vi "readFromXML.vi"(8 "error in (no error)":errorcluster, 10 "XML in":string, 11 "POrigin in":refnum<class "POrigin.lvclass">) -> (0 "error out":errorcluster, 3 "POrigin out":refnum<class "POrigin.lvclass">)   [LabVIEW 2022 SP3, in "TCSDataDefinitions.lvlib" / "TCSCommand.lvlib" / "POriginCommands.lvlib" / "POrigin.lvclass"]
uses:
  POrigin.lvclass
  <userlib>/Common/UnitsAndXML/FlattenItemWithUnitToXML/FlattenLengthToXML/LengthUnit.ctl
  POrigin.lvclass/POrigin.ctl
  POriginCommands/POriginCommands.lvclass
  <userlib>/Common/UnitsAndXML/UnitsAndXML.lvlib
  <userlib>/Common/XML/XMLParser/XMLParser.lvclass
panel:
  out "pOriginY":dbl[unit]
  out "pOriginX":dbl[unit]
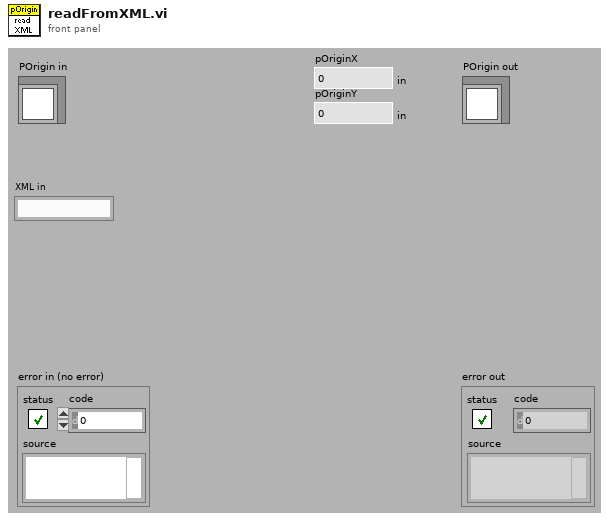
[diagram p1: front panel]
types:
  T1 = typedef "UnitsAndXML.lvlib/LengthUnit.ctl" = enum16{"m", "Angstrom", "AU", "chain", "cm", "cubit", "fathom", "fermi", "ft", "furlong", "hubble", "in", "ly", "mi", "mm", "rod", "um", "yd"}
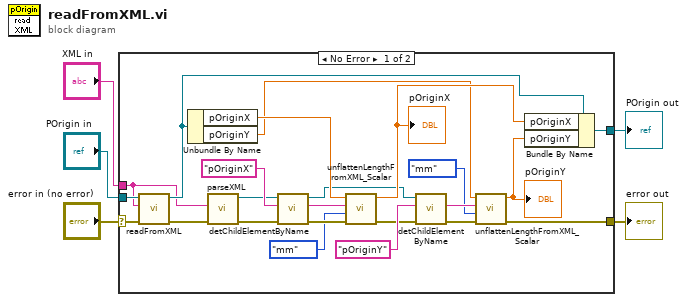
[diagram p0: block diagram]
diagram:
  n1 = case shown="No Error" "error in (no error)" {
    selector: "error in (no error)" -> [w22 w30]
    tunnel: [w8 w30] -> w4
    tunnel: [w25 w29] -> w2
    tunnel: "POrigin in" -> [w24 w29]
    tunnel: "XML in" -> [w20 _]
    frame No Error {
      n2 = call-parent "readFromXML.vi"("error in (no error)"=w22, "XML in"=w20, "POriginCommands in"=w24) -> ("error out"=w21:errorcluster, "POriginCommands out"=w23:refnum<class "POrigin.lvclass">)  [unwired: 7 out]
      n3 = Unbundle By Name(w23) -> ("pOriginX"=w18:dbl[unit], "pOriginY"=w10:dbl[unit])
      n4 = call <userlib>:"parseXML.vi"("error in (no error)"=w21, "XMLString in"=w20) -> ("error out"=w26:errorcluster, "Element out"=w7:refnum<class "XMLParser.lvclass">)  [unwired: 8 in]
      n5 = call <userlib>:"detChildElementByName.vi"("error in (no error)"=w26, "childName"="pOriginX" ("ChildName"), "Element in"=w7) -> ("error out"=w14:errorcluster, "childXML"=w19:string, "Element out"=w6:refnum<class "XMLParser.lvclass">)  [unwired: 5 in, 1 out]
      n6 = call <userlib>:"unflattenLengthFromXML_Scalar.vi"("error in (no error)"=w14, "lengthUnitInXML"=LengthUnit."mm", "xmlString"=w19, "lengthForType"=w18) -> ("error out"=w15:errorcluster, "length"=w17:dbl[unit])  [unwired: 6 in]
      "pOriginX" <- w17
      n7 = call <userlib>:"detChildElementByName.vi"("error in (no error)"=w15, "childName"="pOriginY" ("ChildName"), "Element in"=w6) -> ("error out"=w12:errorcluster, "childXML"=w16:string)  [unwired: 5 in, 2 out]
      n8 = call <userlib>:"unflattenLengthFromXML_Scalar.vi"("error in (no error)"=w12, "lengthUnitInXML"=LengthUnit."mm", "xmlString"=w16, "lengthForType"=w10) -> ("error out"=w8:errorcluster, "length"=w9:dbl[unit])  [unwired: 6 in]
      "pOriginY" <- w9
      n9 = Bundle By Name(cluster=w23, "pOriginX"=w17, "pOriginY"=w9) -> (w25:refnum<class "POrigin.lvclass">)
    }
    frame Error {
    }
  }
  "error out" <- w4
  "POrigin out" <- w2
